vi "K2602 UpdateScript Vsweep.vi"(6 "4-wire":bool, 8 "Script":string, 11 "Settings":T1={"Channel"=enum."Channel A", "Vstart"=-2.0, "Vend"=0.5, "# of points"=30, "NPLC"=1.0, "I compliance"=0.001, "Delay ms"=500.0}) -> (3 "Output":string)   [LabVIEW 2012]
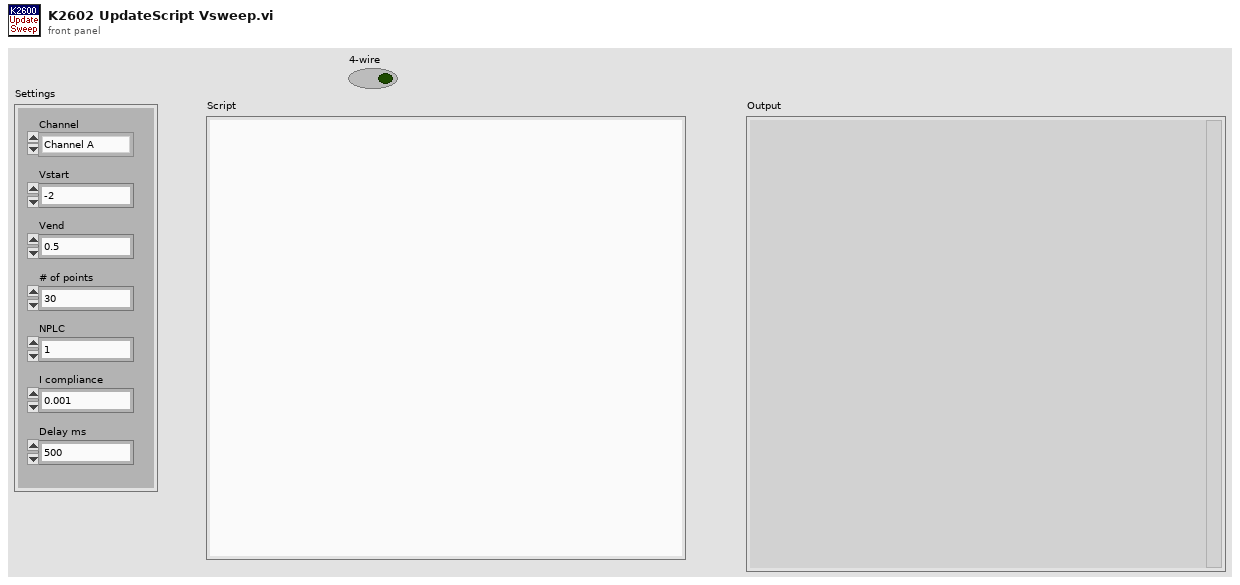
[diagram p1: front panel]
types:
  T1 = cluster{"Channel":enum32{"Channel A", "Channel B"}, "Vstart":dbl, "Vend":dbl, "# of points":u16, "NPLC":dbl, "I compliance":dbl, "Delay ms":dbl}
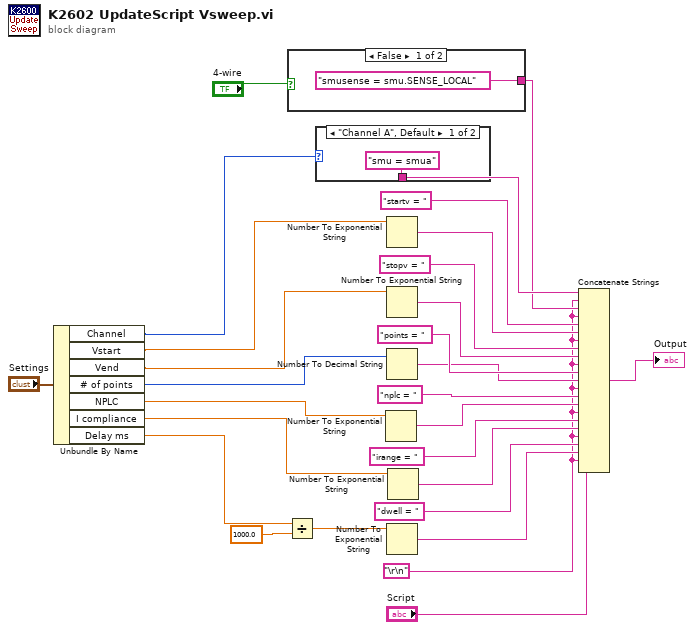
[diagram p0: block diagram]
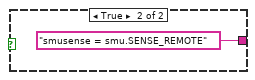
[diagram p2: hidden frame]
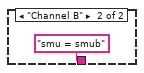
[diagram p3: hidden frame]
diagram:
  w1 = "\r\n"
  n1 = Unbundle By Name("Settings") -> ("Channel"=w16:enum32{"Channel A", "Channel B"}, "Vstart"=w15:dbl, "Vend"=w14:dbl, "# of points"=w13:u16, "NPLC"=w11:dbl, "I compliance"=w7:dbl, "Delay ms"=w10:dbl)
  n2 = Divide(x=w10, y=1000.0) -> (x/y=w18:dbl)
  n3 = case shown="False" "4-wire" {
    tunnel: ["smusense = smu.SENSE_LOCAL" "smusense = smu.SENSE_REMOTE"] -> w2
    frame False {
    }
    frame True {
    }
  }
  n4 = case shown="\"Channel A\", Default" w16 {
    tunnel: ["smu = smua" "smu = smub"] -> w28
    frame "Channel A", Default {
    }
    frame "Channel B" {
    }
  }
  n5 = Number To Exponential String(number=w11) -> (E-format string=w12:string)  [unwired: 3 in]
  n6 = Number To Exponential String(number=w15) -> (E-format string=w26:string)  [unwired: 3 in]
  n7 = Number To Exponential String(number=w14) -> (E-format string=w24:string)  [unwired: 3 in]
  n8 = Number To Decimal String(number=w13) -> (decimal integer string=w22:string)  [unwired: 1 in]
  n9 = Number To Exponential String(number=w18) -> (E-format string=w5:string)  [unwired: 3 in]
  n10 = Number To Exponential String(number=w7) -> (E-format string=w8:string)  [unwired: 3 in]
  n11 = Concatenate Strings(w28, w1, w2, w1, "startv = ", w26, w1, "stopv = ", w24, w1, "points = ", w22, w1, "nplc = ", w12, w1, "irange = ", w8, w1, "dwell = ", w5, w1, "Script") -> (→"Output":string)
